vi "IterationDurationToDt.vi"(11 "Iteration Duration":i64) -> ()   [LabVIEW 2018, in "SubVi.lvlib"]
uses:
  SubVi.lvlib
panel:
  out "dt":dbl
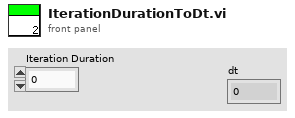
[diagram p1: front panel]
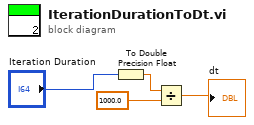
[diagram p0: block diagram]
diagram:
  n1 = To Double Precision Float(number="Iteration Duration") -> (double precision float=w3:dbl)
  n2 = Divide(x=w3, y=1000.0) -> (x/y=→"dt":dbl)
